vi "DriveAnalogGyro_Begin.vi"   [LabVIEW 2023]
uses:
  <vilib>/Rock Robotics/WPI/Gyro/WPI_GyroAnalogOpen.vi
  <vilib>/Rock Robotics/SystemInterfaces/AI/FPGA_AIGyroChannel.ctl
types:
  T1 = typedef "FPGA_AIGyroChannel.ctl" = enum8{"AI 0", "AI 1", "Invalid"}
  T2 = typedef "WPI_GyroDevRef.ctl" = cluster{"DevStatus":errorcluster, "Analog Channel":T3, "Gain (VoltsPerDegree/Second)":dbl, "Gyro Type":enum16{"Analog", "XRS450"}, "Handle":i32, "SPI Bus":T4, "Device Found":bool, "Sample Rate":dbl, "Calibrate On Open":bool, "Offset":dbl}
  T3 = typedef "FPGA_AIChannel.ctl" = enum8{"AI 0", "AI 1", "AI 2", "AI 3", "AI MXP 0", "AI MXP 1", "AI MXP 2", "AI MXP 3", "Invalid"}
  T4 = typedef "spi_bus.ctl" = enum16{"SPI On-Board, CS0", "SPI On-Board, CS1", "SPI On-Board, CS2", "SPI On-Board, CS3", "SPI MXP", "Invalid"}
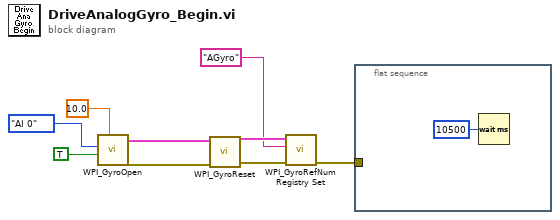
[diagram p0: block diagram]
diagram:
  n1 = call-poly <vilib>:"WPI_GyroOpen.vi"("Calibration Time (s)"=10.0, "Calibrate On Open"=TRUE, "Analog Channel"=FPGA_AIGyroChannel."AI 0") -> ("error out"=w8:errorcluster, "GyroDevRef"=w7:T2)  [unwired: 6 in, 1 out]
  n2 = call <vilib>:"WPI_GyroReset.vi"("error in (no error)"=w8, "GyroDevRef"=w7) -> ("error out"=w6:errorcluster, "GyroDevRef"=w5:T2)  [unwired: 8 in]
  n3 = call <vilib>:"WPI_GyroRefNum Registry Set.vi"("error in (no error)"=w6, "refnum name"="AGyro", "GyroDevRef"=w5) -> ("error out"=w9:errorcluster)  [unwired: 7 in, 1 out]
  n4 = flat-sequence {
    tunnel: w9 -> [_]
    frame #0 {
      n5 = Wait (ms)(milliseconds to wait=u32 10500) -> ()  [unwired: 1 out]
    }
  }
